vi "Prepare folder.vi"(4 "error in":errorcluster, 5 "input main cluster":T1) -> (0 "error out":errorcluster, 1 "output main cluster":T1, 2 "created path":path)   [LabVIEW 2010]
uses:
  Main_cluster.ctl
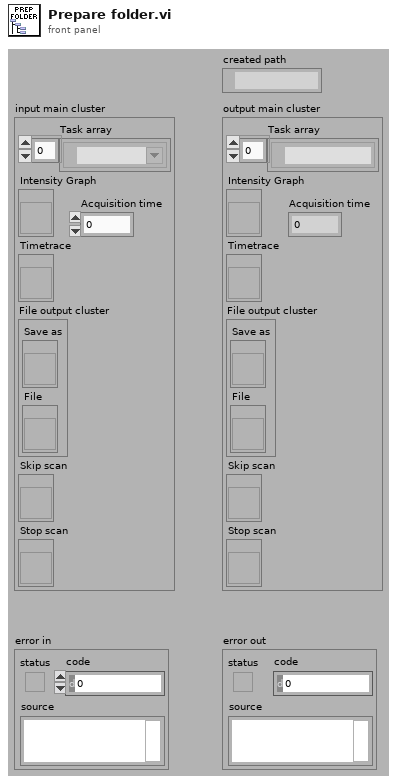
[diagram p1: front panel]
types:
  T1 = typedef "Main_cluster.ctl" = cluster{"Task array":refnum<k21>[], "Intensity Graph":refnum<vi>, "Timetrace":refnum<vi>, "File output cluster":cluster{"Save as":refnum<vi>, "File":refnum<vi>}, "Skip scan":refnum<vi>, "Stop scan":refnum<vi>, "Acquisition time":dbl}
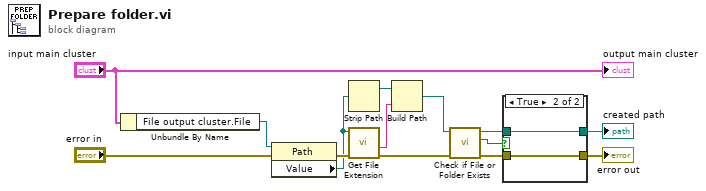
[diagram p0: block diagram]
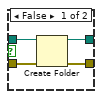
[diagram p2: hidden frame]
diagram:
  n1 = Unbundle By Name("input main cluster") -> ("File output cluster.File"=w11:refnum<vi>)
  n2 = property class="Path"(reference=w11, error in="error in") -> (error out=w13:errorcluster, "Value"=w12:path)  [unwired: 1 out]
  n3 = Strip Path(path=w12) -> (stripped path=w7:path)  [unwired: 1 out]
  n4 = call <vilib>:"Get File Extension.vi"("error in (no error)"=w13, "file"=w12) -> ("error out"=w5:errorcluster, "filename without extension"=w8:string)  [unwired: 6 in, 2 out]
  n5 = Build Path(base path=w7, name or relative path=w8) -> (appended path=w3:path)
  n6 = call <vilib>:"Check if File or Folder Exists.vi"("error in (no error)"=w5, "path"=w3) -> ("error out"=w4:errorcluster, "file or folder exists?"=w2:bool, "dup path"=w1:path)  [unwired: 7 in]
  n7 = case shown="True" w2 {
    tunnel: [w18 w20] -> w10
    tunnel: [w17 w19] -> w9
    tunnel: w4 -> [w16 w19]
    tunnel: w1 -> [w15 w20]
    frame False {
      n8 = Create Folder(path (use dialog)=w15, error in=w16) -> (created path=w18:path, error out=w17:errorcluster)  [unwired: 1 in, 1 out]
    }
    frame True {
    }
  }
  "created path" <- w10
  "error out" <- w9
  "output main cluster" <- "input main cluster"
